vi "Main.vi"() -> ()   [LabVIEW 2021]
doc: "The myRIO Project template acquires acceleration data from the onboard accelerometer and displays the changes of acceleration values in a waveform chart."
uses:
  <vilib>/myRIO/Instrument Drivers/Onboard IO/AI/typedefs/AI Reference.ctl
  <vilib>/myRIO/Common/Instrument Driver Framework/Utilities/typedefs/myRIO Generic Hardware Reference.ctl
  <vilib>/myRIO/Common/Instrument Driver Framework/Utilities/typedefs/Hardware Version Enum.ctl
  <vilib>/myRIO/Common/Instrument Driver Framework/Utilities/typedefs/myRIO v1.0 Reference.ctl
  <vilib>/myRIO/Common/Instrument Driver Framework/Utilities/typedefs/Generic FPGA Reference.ctl
  <vilib>/myRIO/Common/Instrument Driver Framework/myRIO v1.0/AI/typedefs/AI Channels List.ctl
  <vilib>/myRIO/Common/Instrument Driver Framework/myRIO v1.0/AI/typedefs/AI Channels Enum.ctl
  <vilib>/myRIO/Common/Instrument Driver Framework/Utilities/typedefs/Analog Scaling Constants List.ctl
  <vilib>/myRIO/Common/Instrument Driver Framework/Utilities/typedefs/Analog Scaling Constants.ctl
  <vilib>/userDefined/High Color/nirio_resource_hc.ctl
  <vilib>/myRIO/Instrument Drivers/Onboard IO/PWM/typedefs/PWM Reference.ctl
  <vilib>/myRIO/Common/Instrument Driver Framework/myRIO v1.0/PWM/typedefs/PWM Channels Enum.ctl
  <vilib>/myRIO/Instrument Drivers/Onboard IO/PWM/typedefs/PWM Configuration.ctl
  <vilib>/myRIO/Common/Instrument Driver Framework/Utilities/vis/Is FPGA Ref Available.vi
  <vilib>/myRIO/Common/Instrument Driver Framework/myRIO v1.0/AI/vis/myRIO v1.1 Open AI.vi
  <vilib>/myRIO/Instrument Drivers/Onboard IO/AI/vis/Read.vi
  <vilib>/myRIO/Common/Instrument Driver Framework/myRIO v1.0/PWM/vis/myRIO v1.1 Open PWM.vi
  <vilib>/myRIO/Instrument Drivers/Onboard IO/PWM/vis/Set Duty Cycle and Frequency.vi
  <vilib>/myRIO/Common/Instrument Driver Framework/Utilities/vis/Validate Channels.vi
  <vilib>/myRIO/Common/Instrument Driver Framework/myRIO v1.0/AI/vis/myRIO v1.0 Reserve AI.vi
  <vilib>/myRIO/Common/Instrument Driver Framework/myRIO v1.0/PWM/vis/myRIO v1.0 Reserve PWM.vi
  <vilib>/myRIO/Common/Instrument Driver Framework/myRIO v1.0/UART/vis/myRIO v1.0 Close UART.vi
  <vilib>/myRIO/Common/Instrument Driver Framework/myRIO v1.0/AI/vis/myRIO v1.0 Build MUX Configuration AI.vi
  <vilib>/myRIO/Common/Instrument Driver Framework/myRIO v1.0/Resource Manager/vis/myRIO v1.0 Reserve Channel List.vi
  <vilib>/myRIO/Common/Instrument Driver Framework/myRIO v1.0/PWM/vis/myRIO v1.0 Build MUX Configuration PWM.vi
  <vilib>/myRIO/Common/Instrument Driver Framework/myRIO v1.0/Resource Manager/vis/myRIO v1.0 Reserve Channel.vi
  <vilib>/myRIO/Common/Instrument Driver Framework/myRIO v1.0/Resource Manager/vis/myRIO v1.0 Unreserve Channel.vi
  <vilib>/myRIO/Common/Instrument Driver Framework/myRIO v1.0/Resource Manager/vis/myRIO v1.0 Create Configuration List.vi
  <vilib>/myRIO/Common/Instrument Driver Framework/myRIO v1.0/Resource Manager/vis/myRIO v1.0 Build Mutex Name.vi
  <vilib>/Utility/VariantDataType/GetNumericInfo.vi
  <vilib>/Utility/error.llb/Error Cluster From Error Code.vi
  <vilib>/myRIO/Common/Instrument Driver Framework/myRIO v1.0/myRIO v1.1 Open.vi
  <vilib>/myRIO/Common/Instrument Driver Framework/myRIO v1.0/AI/vis/myRIO v1.0 Get Scaling Constants AI.vi
  <vilib>/myRIO/Common/Instrument Driver Framework/Utilities/vis/IO Manager.vi
  <vilib>/myRIO/Common/Instrument Driver Framework/Utilities/vis/Configuration Manager.vi
  <vilib>/myRIO/Common/Instrument Driver Framework/myRIO v1.0/myRIO v1.0 Close.vi
  <vilib>/myRIO/Common/Instrument Driver Framework/myRIO v1.0/AI/vis/myRIO v1.0 Read AI.vi
  <vilib>/myRIO/Common/Instrument Driver Framework/myRIO v1.0/Resource Manager/vis/myRIO v1.0 Configure IO.vi
  <vilib>/myRIO/Common/Instrument Driver Framework/myRIO v1.0/PWM/vis/myRIO v1.0 Write PWM.vi
  <vilib>/myRIO/Common/Instrument Driver Framework/Utilities/vis/FPGA Ref Manager.vi
  <vilib>/myRIO/Common/Instrument Driver Framework/myRIO v1.0/myRIO v1.0 Reset FPGA.vi
  <vilib>/myRIO/Common/Instrument Driver Framework/myRIO v1.0/IRQ/vis/myRIO v1.0 IRQ Info FGV.vi
  <vilib>/myRIO/Common/Instrument Driver Framework/myRIO v1.0/IRQ/vis/myRIO v1.0 Timer IRQ Info FGV.vi
  <vilib>/myRIO/Common/Instrument Driver Framework/myRIO v1.0/IRQ/vis/myRIO v1.0 ISR Agent.vi
  <vilib>/myRIO/Instrument Drivers/Utilities/vis/Reset Index.vi
  <vilib>/myRIO/Common/Instrument Driver Framework/myRIO v1.0/Resource Manager/vis/myRIO v1.0 Block Write Resource Manager.vi
  <vilib>/myRIO/Express VI/Onboard IO/AI/AI Express VI.xnode
  <vilib>/myRIO/Instrument Drivers/Onboard IO/AI/vis/myRIO AI Open.xnode
  <vilib>/myRIO/Express VI/Onboard IO/PWM/PWM Express VI.xnode
  <vilib>/myRIO/Instrument Drivers/Onboard IO/PWM/vis/myRIO PWM Open.xnode
  <vilib>/myRIO/Instrument Drivers/Onboard IO/AI/AI.lvlib
  <vilib>/myRIO/Instrument Drivers/Onboard IO/PWM/PWM.lvlib
  <vilib>/myRIO/Instrument Drivers/Utilities/Utilities.lvlib
panel:
  out "Feedback":dbl
  out "Raw Feedback":dbl format="%#_2g"
  out "Raw Set Point":dbl format="%#.2g"
  in  "Actuator":bool
  in  "Right Feedback Limit":dbl
  in  "Left Feedback Limit":dbl
  in  "Right Set Point Limit":dbl
  in  "Left Set Point Limit":dbl
  out "Waveform Chart":cluster{"t":dbl, dbl, dbl, dbl}(graph)
  out "Position (Degree)":dbl(knob) scale=-45.0..45.0 scale format="%#_2g"
  out "Position (Voltage)":dbl(knob) scale=0.0..5.0 scale format="%#_2g"
  in  "D EN":bool
  in  "I EN":bool
  in  "P EN":bool
  in  "Stop Button":bool
  out "Derivative":dbl format="%#_2g"
  out "Integral":dbl format="%#_2g"
  out "Proportional":dbl format="%#_2g"
  out "Error":dbl format="%#_2g"
  out "Set Point":dbl format="%#_2g"
  in  "Kd":dbl
  in  "Ki":dbl
  in  "Kp":dbl
  out "error out":errorcluster
  # "Seesaw with PID Contoller\nInstructions:\n1. Check the myRIO target IP address in the project and make sure the target IP address is correct. \n2. Check limit of set point and feedback voltage range.\n3. Specify limit parameter.\n4. Run this VI."
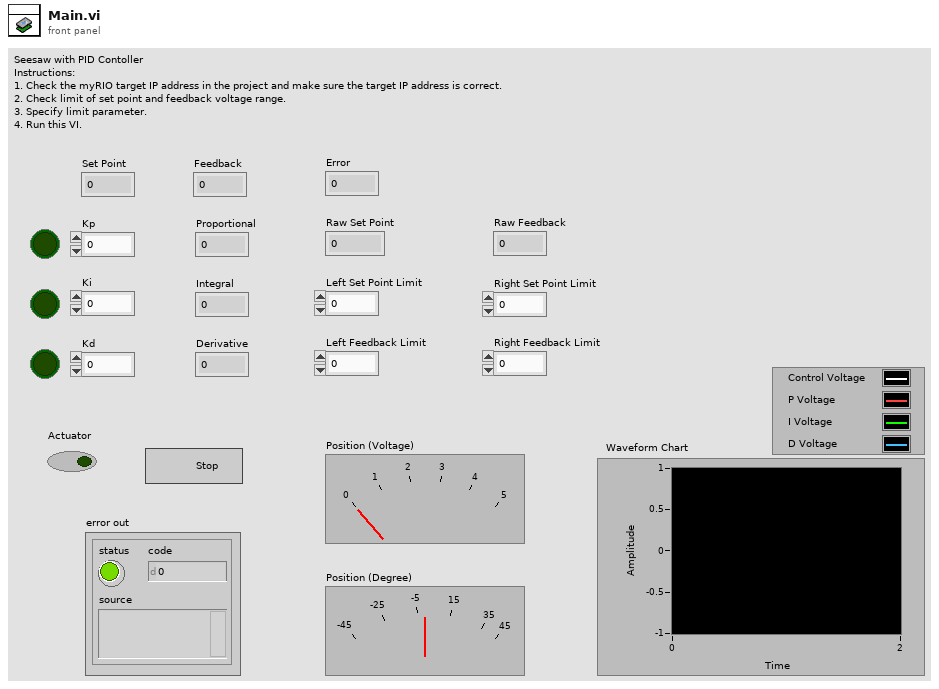
[diagram p1: front panel]
types:
  T1 = typedef "AI.lvlib/AI Reference.ctl" = cluster{"myRIO Reference":T2, "AI Channels List":T6, "AI Scaling Constants List":T8}
  T2 = typedef "myRIO Generic Hardware Reference.ctl" = cluster{"myRIO Model":T3, "myRIO Hardware Reference":T4}
  T3 = typedef "Hardware Version Enum.ctl" = enum16{"Unknown", "myRIO-1900", "myRIO-1950", "roboRIO", "NI ELVIS RIO CM", "ELVIS III"}
  T4 = typedef "myRIO v1.0 Reference.ctl" = cluster{"Generic FPGA Reference":T5, "Allow multiple opens":bool}
  T5 = typedef "Generic FPGA Reference.ctl" = refnum<k20>
  T6 = typedef "AI Channels List.ctl" = T7[]
  T7 = typedef "AI Channels Enum.ctl" = enum16{"Not Connected", "AudioIn/Left", "AudioIn/Right", "C/AI0", "C/AI1", "A/AI0", "A/AI1", "A/AI2", "A/AI3", "A/AI4", "A/AI5", "A/AI6", "A/AI7", "B/AI0", "B/AI1", "B/AI2", "B/AI3", "B/AI4", "B/AI5", "B/AI6", "B/AI7", "AI/AI0", "AI/AI1", "AI/AI2", "AI/AI3", "A/AI0 (DIFF)", "A/AI1 (DIFF)", "A/AI2 (DIFF)", "A/AI3 (DIFF)", "B/AI0 (DIFF)", "B/AI1 (DIFF)", "B/AI2 (DIFF)", "B/AI3 (DIFF)"}
  T8 = typedef "Analog Scaling Constants List.ctl" = T9[]
  T9 = typedef "Analog Scaling Constants.ctl" = cluster{"LSB Weight (Volts)":dbl, "Offset (Volts)":dbl, "Signed?":bool}
  T10 = typedef "nirio_resource_hc.ctl" = tag
  T11 = typedef "PWM.lvlib/PWM Reference.ctl" = cluster{"myRIO Reference":T2, "PWM Channels Enum":T12, "PWM Configuration":T13}
  T12 = typedef "PWM Channels Enum.ctl" = enum16{"Not Connected", "C/PWM0", "C/PWM1", "A/PWM0", "A/PWM1", "A/PWM2", "A/PWM3", "A/PWM4", "A/PWM5", "A/PWM6", "A/PWM7", "A/PWM8", "A/PWM9", "A/PWM10", "A/PWM11", "A/PWM12", "A/PWM13", "A/PWM14", "A/PWM15", "A/PWM16", "A/PWM17", "A/PWM18", "A/PWM19", "B/PWM0", "B/PWM1", "B/PWM2", "B/PWM3", "B/PWM4", "B/PWM5", "B/PWM6", "B/PWM7", "B/PWM8", "B/PWM9", "B/PWM10", "B/PWM11", "B/PWM12", "B/PWM13", "B/PWM14", "B/PWM15", "B/PWM16", "B/PWM17", "B/PWM18", "B/PWM19", "PWM/PWM0", "PWM/PWM1", "PWM/PWM2", "PWM/PWM3", "PWM/PWM4", "PWM/PWM5", "PWM/PWM6", "PWM/PWM7", "PWM/PWM8", "PWM/PWM9"}
  T13 = typedef "PWM.lvlib/PWM Configuration.ctl" = cluster{"Frequency":dbl, "Duty Cycle":dbl}
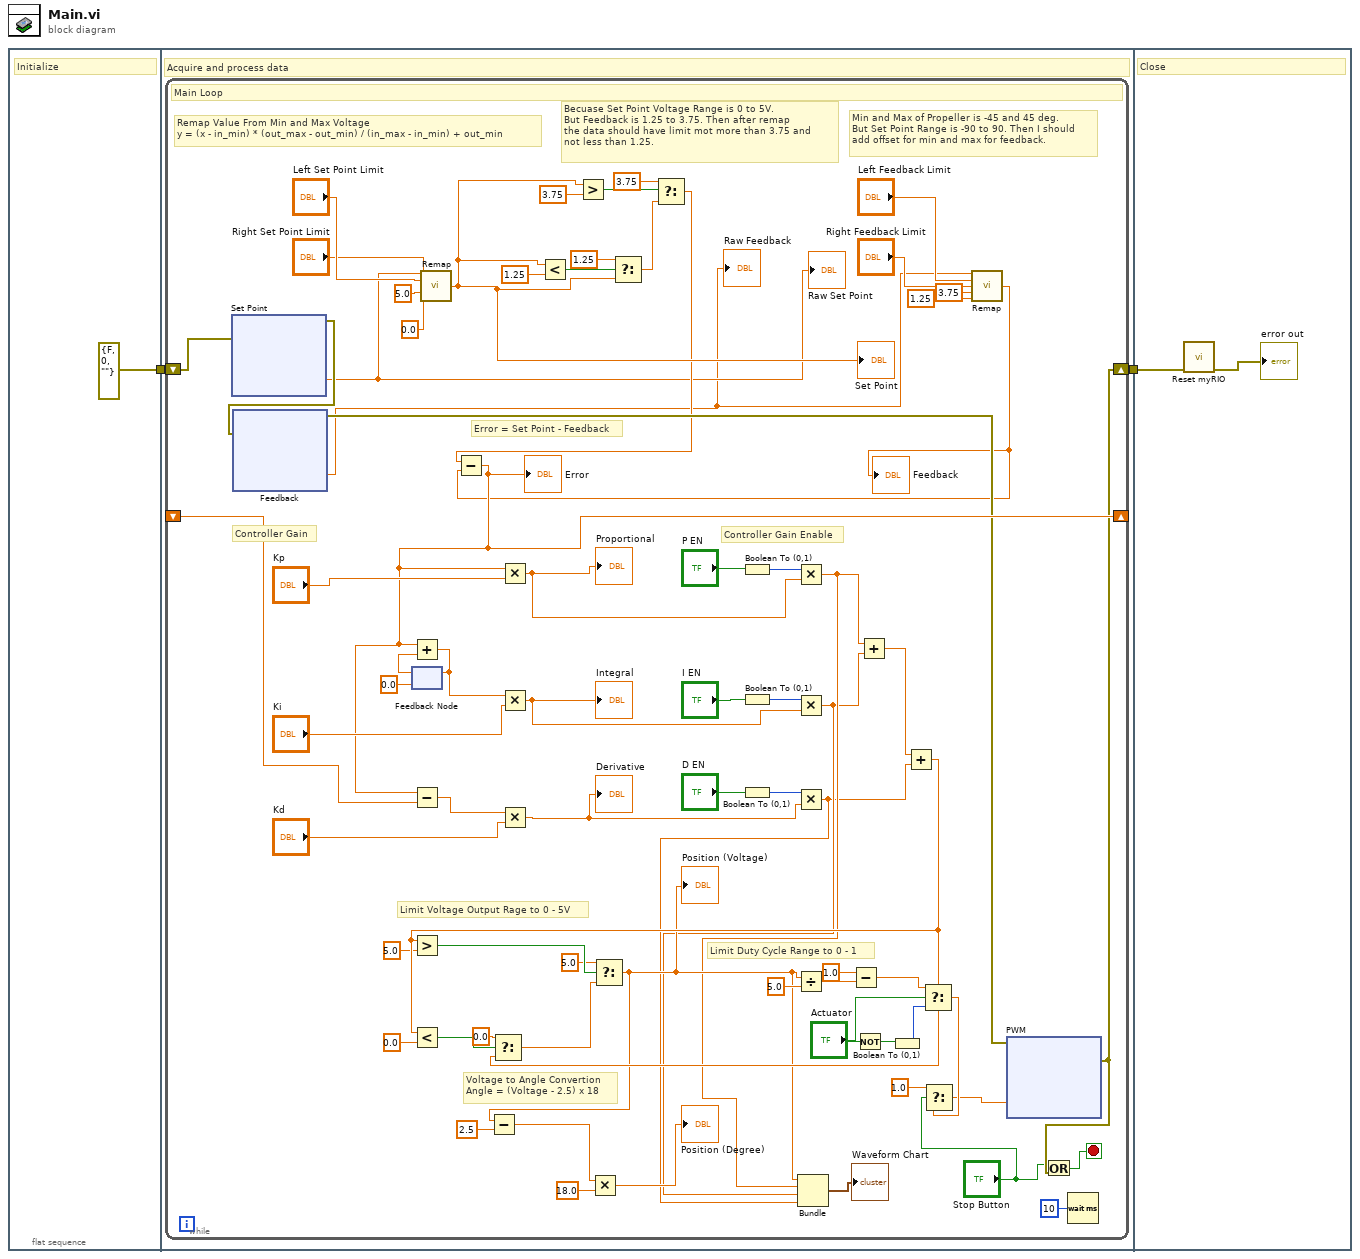
[diagram p0: block diagram]
diagram:
  n1 = flat-sequence {
    tunnel: [errorcluster {"status"=FALSE, "code"=0, "source"=""} ("error in (no error)")] -> w2
    tunnel: w2 -> [w5]
    tunnel: [w4] -> w1
    tunnel: w1 -> [w188]
    frame #0 {
      # "Initialize"
    }
    frame #1 {
      # "Acquire and process data"
      n2 = while {
        shift-right: [w11] -> w4
        shift-left: w5 -> [w78]
        shift-right: [w71] -> _
        shift-left: _ -> [w72]
        stop <- w27 stop-if-true
        # "Becuase Set Point Voltage Range is 0 to 5V.\nBut Feedback is 1.25 to 3.75. Then after remap\nthe data should have limit mot more than 3.75 and\nnot less than 1.25."
        # "Min and Max of Propeller is -45 and 45 deg. \nBut Set Point Range is -90 to 90. Then I should \nadd offset for min and max for feedback."
        # "Remap Value From Min and Max Voltage\ny = (x - in_min) * (out_max - out_min) / (in_max - in_min) + out_min"
        # "Controller Gain Enable"
        # "Error = Set Point - Feedback"
        # "Controller Gain"
        # "Limit Duty Cycle Range to 0 - 1"
        # "Limit Voltage Output Rage to 0 - 5V"
        # "Voltage to Angle Convertion\nAngle = (Voltage - 2.5) x 18"
        # "Main Loop"
        n3 = xnode "Set Point"("error in (no error)"=w78) -> ("A/AI0 (Pin 3)"=w26:dbl, "error out"=w52:errorcluster)
        "Raw Set Point" <- w26
        n4 = xnode "Feedback"("error in (no error)"=w52) -> ("A/AI1 (Pin 5)"=w25:dbl, "error out"=w51:errorcluster)
        "Raw Feedback" <- w25
        n5 = feedback #1(0.0) -> (w76:dbl)
        n6 = call "Remap.vi"("x"=w26, "In Min"="Left Set Point Limit", "In Max"="Right Set Point Limit", "Out Min"=5.0, "Out Max"=0.0) -> ("y"=w29:dbl)  [unwired: 10 in]
        "Set Point" <- w29
        n7 = Less?(x=w29, y=1.25) -> (x < y?=w32:bool)
        n8 = Greater?(x=w29, y=3.75) -> (0:w35:bool)
        n9 = Select(t=1.25, s=w32, f=w29) -> (s? t:f=w33:dbl)
        n10 = Select(t=3.75, s=w35, f=w33) -> (s? t:f=w28:dbl)
        n11 = Boolean To (0,1)(Boolean="P EN") -> (0, 1=w67:i16)
        n12 = Boolean To (0,1)(Boolean="I EN") -> (0, 1=w65:i16)
        n13 = Boolean To (0,1)(Boolean="D EN") -> (0, 1=w63:i16)
        n14 = Not(x="Actuator") -> (.not. x?=w22:bool)
        n15 = Boolean To (0,1)(Boolean=w22) -> (0, 1=w20:i16)
        n16 = call "Remap.vi"("x"=w25, "In Min"="Left Feedback Limit", "In Max"="Right Feedback Limit", "Out Min"=3.75, "Out Max"=1.25) -> ("y"=w12:dbl)  [unwired: 10 in]
        "Feedback" <- w12
        n17 = Subtract(x=w28, y=w12) -> (x-y=w71:dbl)
        "Error" <- w71
        n18 = Add(x=w71, y=w76) -> (x+y=w74:dbl)
        n19 = feedback-in #1(w74) -> ()
        n20 = Subtract(x=w71, y=w72) -> (x-y=w70:dbl)
        n21 = Multiply(x=w71, y="Kp") -> (x*y=w18:dbl)
        "Proportional" <- w18
        n22 = Multiply(x=w74, y="Ki") -> (x*y=w17:dbl)
        "Integral" <- w17
        n23 = Multiply(x=w70, y="Kd") -> (x*y=w16:dbl)
        "Derivative" <- w16
        n24 = Multiply(x=w67, y=w18) -> (x*y=w15:dbl)
        n25 = Multiply(x=w65, y=w17) -> (x*y=w14:dbl)
        n26 = Multiply(x=w63, y=w16) -> (x*y=w13:dbl)
        n27 = Add(x=w15, y=w14) -> (x+y=w62:dbl)
        n28 = Add(x=w62, y=w13) -> (x+y=w57:dbl)
        n29 = Greater?(x=w57, y=5.0) -> (0:w61:bool)
        n30 = Less?(x=w57, y=0.0) -> (x < y?=w60:bool)
        n31 = Select(t=0.0, s=w60, f=w57) -> (s? t:f=w59:dbl)
        n32 = Select(t=5.0, s=w61, f=w59) -> (s? t:f=w46:dbl)
        "Position (Voltage)" <- w46
        n33 = Subtract(x=w46, y=2.5) -> (x-y=w50:dbl)
        n34 = Multiply(x=w50, y=18.0) -> (x*y=→"Position (Degree)":dbl)
        n35 = Divide(x=w46, y=5.0) -> (x/y=w23:dbl)
        n36 = Bundle("t"=w46, w15, w14, w13) -> (→"Waveform Chart":cluster{"t":dbl, dbl, dbl, dbl})  [unwired: 1 in]
        n37 = Subtract(x=1.0, y=w23) -> (x-y=w21:dbl)
        n38 = Select(t=w21, s="Actuator", f=w20) -> (s? t:f=w9:dbl)
        n39 = Select(t=1.0, s="Stop Button", f=w9) -> (s? t:f=w8:dbl)
        n40 = xnode "PWM"("Duty Cycle"=w8, "error in (no error)"=w51) -> ("error out"=w11:errorcluster)
        n41 = Or(x="Stop Button", y=w11) -> (x .or. y?=w27:bool)
        n42 = Wait (ms)(milliseconds to wait=u32 10) -> ()  [unwired: 1 out]
      }
    }
    frame #2 {
      # "Close"
      n43 = call <vilib>:"Reset myRIO.vi"("error in (no error)"=w188) -> ("error out"=→"error out":errorcluster)  [unwired: 10 in]
    }
  }
